vi "mouseSignals.vi"() -> ()   [LabVIEW 2024]
uses:
  <vilib>/Utility/inputDevices.llb/mouseAcquire.vi
panel:
  in  "stop":bool
  out "Scrolling":i32
  out "button 2":bool
  out "button 3":bool
  out "button 4":bool
  out "button 1":bool
  out "Vertical":i32
  out "Horizontal":i32
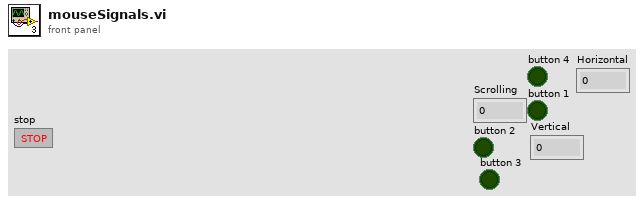
[diagram p1: front panel]
types:
  T1 = cluster{"Horizontal":i32, "Vertical":i32, "Scrolling":i32}
  T2 = cluster{"button 1":bool, "button 2":bool, "button 3":bool, "button 4":bool}
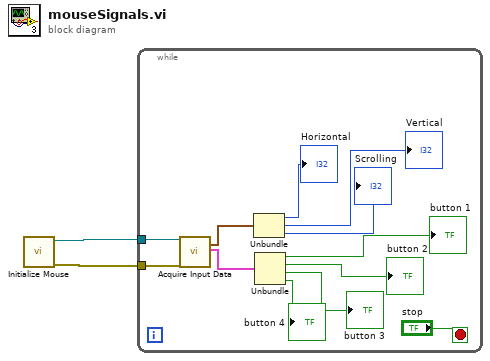
[diagram p0: block diagram]
diagram:
  n1 = call <vilib>:"Initialize Mouse.vi"() -> ("error out"=w1:errorcluster, "device ID"=w2:refnum<k1>)  [unwired: 10 in]
  n2 = while {
    tunnel: w2 -> [w14]
    tunnel: w1 -> [w13]
    stop <- "stop" stop-if-true
    n3 = call-poly <vilib>:"Acquire Input Data.vi"("device ID"=w14, "error in (no error)"=w13) -> ("axis info"=w11:T1, "button info"=w12:T2)  [unwired: 14 in, 2 out]
    n4 = Unbundle(w11) -> ("Horizontal"=→"Horizontal":i32, "Vertical"=→"Vertical":i32, "Scrolling"=→"Scrolling":i32)
    n5 = Unbundle(w12) -> ("button 1"=→"button 1":bool, "button 2"=→"button 2":bool, "button 3"=→"button 3":bool, "button 4"=→"button 4":bool)
  }
